vi "Concatenate PDF Standalone.vi"(0 "New File name":path, 7 "PDF Files  to concatenate [ ]":T1[](array[typedef]), 11 "error in (no error)":errorcluster) -> (15 "error out":errorcluster)   [LabVIEW 2019, in "Exaprom PDF.lvlib"]
doc: "Standalone.\n\nVersion 2.0\nDeveloped by Jean-Marc Simard\nCopyright © 2012, Exaprom Inc.\nAll rights reserved.\nLicense: BSD\n\nWith iTextSharp Library"
uses:
  Controls/Concatenate Controls/PDF file to concatenate.ctl
  Controls/General Controls/Create or close.ctl
  Controls/Concatenate Controls/PDF File and position.ctl
  Controls/Concatenate Controls/PDF file source.ctl
  Exaprom PDF.lvlib
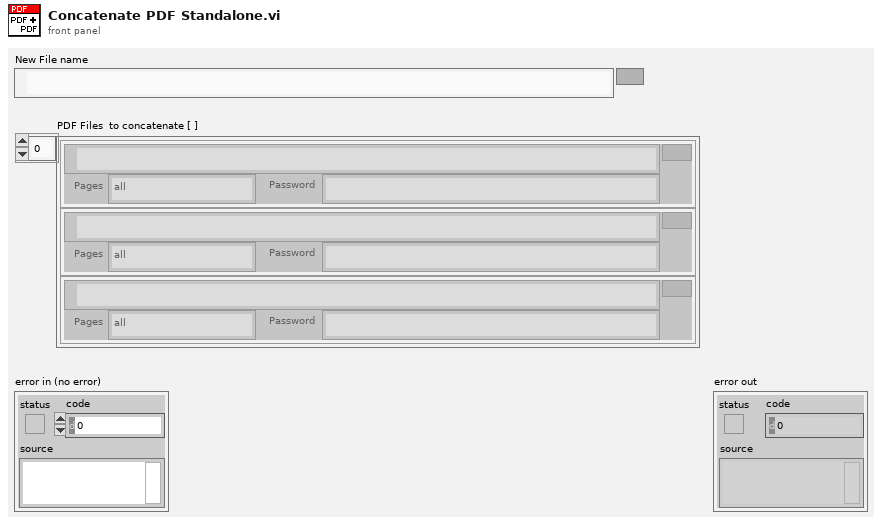
[diagram p1: front panel]
types:
  T1 = typedef "Exaprom PDF.lvlib/PDF file to concatenate.ctl" = cluster{"Path":path, "Pages":string, "Password":string}
  T2 = typedef "Exaprom PDF.lvlib/Create or close.ctl" = enum16{"Create", "Close"}
  T3 = typedef "Exaprom PDF.lvlib/PDF File and position.ctl" = cluster{"Path":path, "Pages":string, "Source":T4, "Start at page old":i32, "Start at page new":i32, "Owner password":string}
  T4 = typedef "Exaprom PDF.lvlib/PDF file source.ctl" = enum16{"PDF Report", "File to add"}
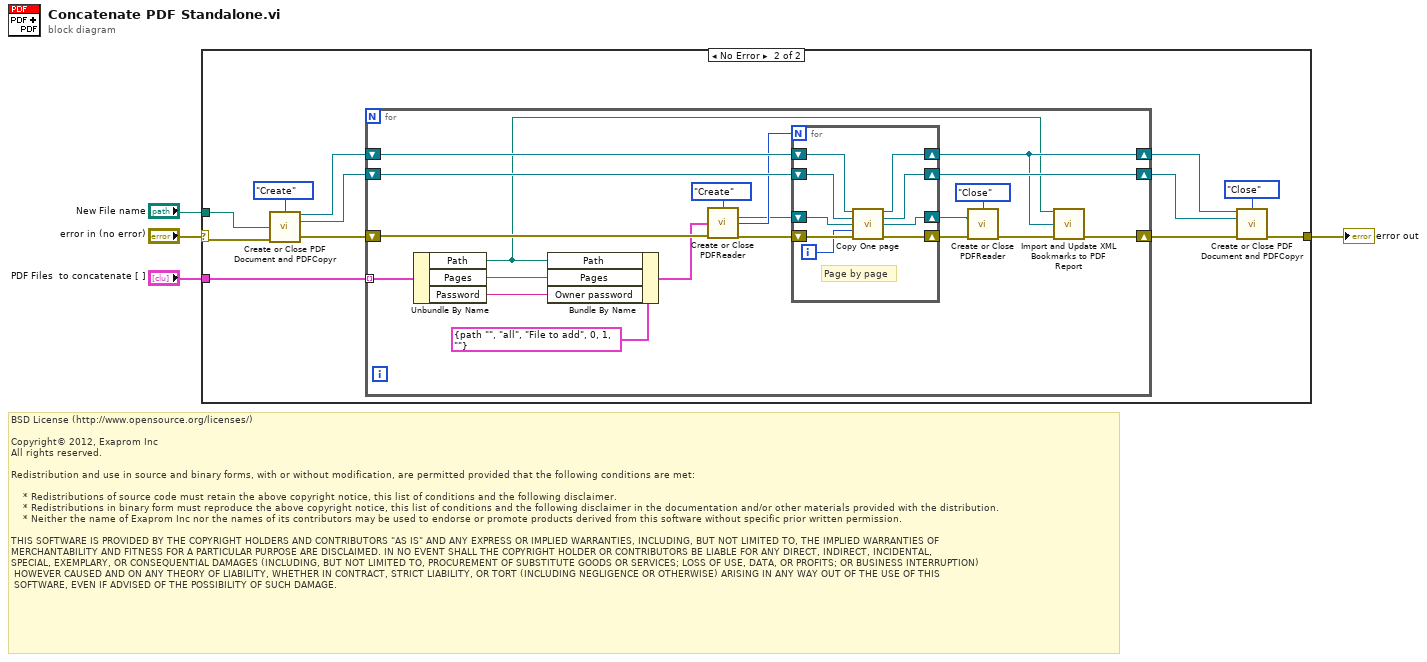
[diagram p0: block diagram]
diagram:
  # "BSD License (http://www.opensource.org/licenses/)\n\nCopyright© 2012, Exaprom Inc\nAll rights reserved.\n\nRedistribution and use in source and binary forms, with or without modification, are permitted provided that the following conditions are met:\n\n    * Redistributions of source code must retain the above copyright notice, this list of conditions and the following disclaimer.\n    * Redistributions in binary form must reproduce the above copyright notice, this list of conditions and the following disclaimer in the documentation and/or other materials provided with the distribution.\n    * Neither the name of Exaprom Inc nor the names of its contributors may be used to endorse or promote products derived from this software without specific prior written permission.\n\nTHIS SOFTWARE IS PROVIDED BY THE COPYRIGHT HOLDERS AND CONTRIBUTORS \"AS IS\" AND ANY EXPRESS OR IMPLIED WARRANTIES, INCLUDING, BUT NOT LIMITED TO, THE IMPLIED WARRANTIES OF \nMERCHANTABILITY AND FITNESS FOR A PARTICULAR PURPOSE ARE DISCLAIMED. IN NO EVENT SHALL THE COPYRIGHT HOLDER OR CONTRIBUTORS BE LIABLE FOR ANY DIRECT, INDIRECT, INCIDENTAL,\nSPECIAL, EXEMPLARY, OR CONSEQUENTIAL DAMAGES (INCLUDING, BUT NOT LIMITED TO, PROCUREMENT OF SUBSTITUTE GOODS OR SERVICES; LOSS OF USE, DATA, OR PROFITS; OR BUSINESS INTERRUPTION)\n HOWEVER CAUSED AND ON ANY THEORY OF LIABILITY, WHETHER IN CONTRACT, STRICT LIABILITY, OR TORT (INCLUDING NEGLIGENCE OR OTHERWISE) ARISING IN ANY WAY OUT OF THE USE OF THIS\n SOFTWARE, EVEN IF ADVISED OF THE POSSIBILITY OF SUCH DAMAGE."
  n1 = case shown="No Error" "error in (no error)" {
    selector: "error in (no error)" -> [w5 w15]
    tunnel: [w5 w9] -> w4
    tunnel: "New File name" -> [_ w12]
    tunnel: "PDF Files  to concatenate [ ]" -> [_ w17]
    frame Error {
    }
    frame No Error {
      n2 = call "Create or Close PDF Document and PDFCopyr.vi"("Action"=Create_or_close."Create", "File name"=w12, "error in (no error)"=w15) -> ("PDF Copy OUT"=w14:refnum<k24>, "PDF Document OUT"=w13:refnum<k24>, "error out"=w16:errorcluster)  [unwired: 10 in]
      n3 = for {
        tunnel: w17 -> [w26] mode=indexing
        shift-right: [w35] -> w7
        shift-left: w13 -> [w37]
        shift-right: [w20] -> w10
        shift-left: w16 -> [w33]
        shift-right: [w19] -> w8
        shift-left: w14 -> [w36]
        n4 = Unbundle By Name(w26) -> ("Path"=w18:path, "Pages"=w24:string, "Password"=w22:string)
        n5 = Bundle By Name(cluster=T3 {"Path"=path "", "Pages"="all", "Source"=enum."File to add", "Start at page old"=0, "Start at page new"=1, "Owner password"=""} ("PDF File and position"), "Path"=w18, "Pages"=w24, "Owner password"=w22) -> (w23:T3)
        n6 = call "Create or Close PDFReader.vi"("Action"=Create_or_close."Create", "PDF File and position"=w23, "error in (no error)"=w33) -> ("PdfReader OUT"=w31:refnum<k24>, "NumberOfPages"=w32:i32, "error out"=w34:errorcluster)  [unwired: 8 in, 2 out]
        n7 = for {
          N: w32 -> [_]
          shift-right: [w40] -> w35
          shift-left: w37 -> [w44]
          shift-right: [w39] -> w29
          shift-left: w31 -> [w45]
          shift-right: [w38] -> w30
          shift-left: w34 -> [w46]
          shift-right: [w41] -> w19
          shift-left: w36 -> [w43]
          i -> [w42]
          # "Page by page"
          n8 = call "Copy One page.vi"("PDFCopy IN"=w43, "PDF Document IN"=w44, "PdfReader IN"=w45, "index"=w42, "error in (no error)"=w46) -> ("PDFCopy OUT"=w41:refnum<k24>, "PDF Document OUT"=w40:refnum<k24>, "PdfReader OUT"=w39:refnum<k24>, "error out"=w38:errorcluster)  [unwired: 6 in, 1 out]
        }
        n9 = call "Create or Close PDFReader.vi"("Action"=Create_or_close."Close", "PdfReader IN"=w29, "error in (no error)"=w30) -> ("error out"=w21:errorcluster)  [unwired: 8 in, 4 out]
        n10 = call "Import and Update XML Bookmarks to PDF Report.vi"("PDF path file"=w18, "PDFCopy"=w19, "error in (no error)"=w21) -> ("error out"=w20:errorcluster)  [unwired: 12 in]
      }
      n11 = call "Create or Close PDF Document and PDFCopyr.vi"("PDF Copy IN"=w8, "Action"=Create_or_close."Close", "PDF Document IN"=w7, "error in (no error)"=w10) -> ("error out"=w9:errorcluster)  [unwired: 9 in, 2 out]
    }
  }
  "error out" <- w4
